vi "Unload Theme-Root Only.vi"(8 "Error In":errorcluster, 11 "Appearance Actor in":refnum<class "Appearance Actor.lvclass">) -> (0 "Error Out":errorcluster, 3 "Appearance Actor out":refnum<class "Appearance Actor.lvclass">)   [LabVIEW 2021, in "Appearance Actor.lvlib" / "Appearance Actor.lvclass"]
uses:
  Appearance Actor.lvclass
  C:/Program Files (x86)/National Instruments/LabVIEW 2021/vi.lib/ActorFramework/Actor/Actor.lvclass
  <vilib>/ActorFramework/Message Enqueuer/Message Enqueuer.lvclass
  <vilib>/ActorFramework/Actor/Actor.lvclass/Actor.ctl
  Appearance Actor.lvclass/Appearance Actor.ctl
  <vilib>/Utility/config.llb/Config Data RefNum.ctl
  <vilib>/ActorFramework/Actor/Actor.lvclass
  <vilib>/Utility/config.llb/NI_LVConfig.lvlib
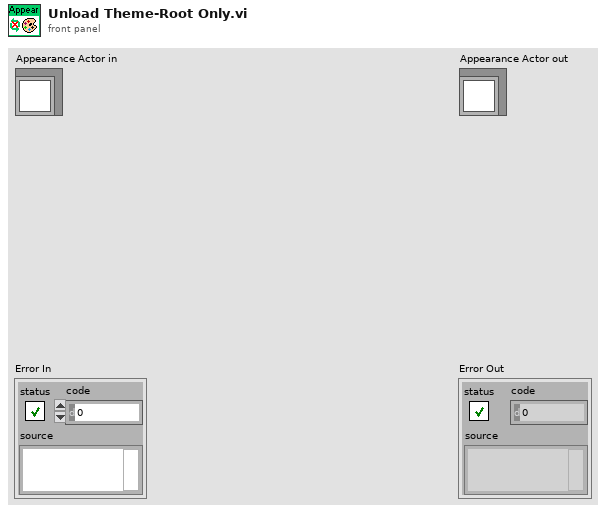
[diagram p1: front panel]
types:
  T1 = typedef "NI_LVConfig.lvlib/Config Data RefNum.ctl" = refnum<k1>
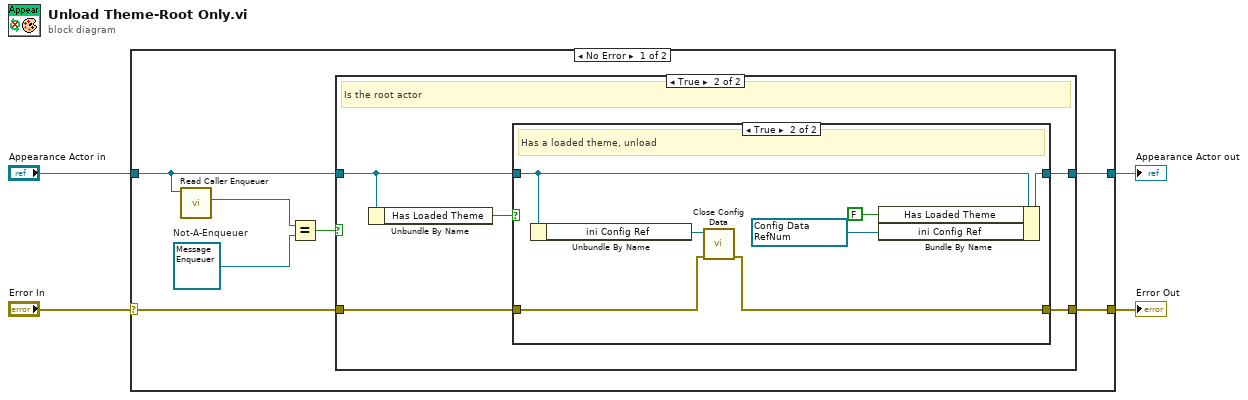
[diagram p0: block diagram]
diagram:
  n1 = case shown="No Error" "Error In" {
    selector: "Error In" -> [w6 w29]
    tunnel: [w5 w29] -> w3
    tunnel: [w7 w28] -> w1
    tunnel: "Appearance Actor in" -> [w8 w28]
    frame No Error {
      w10 = refnum<class "Message Enqueuer.lvclass"> refnum  # Not-A-Enqueuer
      n2 = call <vilib>:"Read Caller Enqueuer.vi"("Actor"=w8) -> ("Caller Enqueuer"=w11:refnum<class "Message Enqueuer.lvclass">)  [unwired: 10 in]
      n3 = Equal?(x=w11, y=w10) -> (x = y?=w9:bool)
      n4 = case shown="True" w9 {
        tunnel: w6 -> [w12 w17]
        tunnel: [w12 w16] -> w5
        tunnel: [w13 w18] -> w7
        tunnel: w8 -> [w13 w15]
        frame False {
          # "Is a nested actor"
        }
        frame True {
          # "Is the root actor"
          n5 = Unbundle By Name(w15) -> ("Has Loaded Theme"=w14:bool)
          n6 = case shown="True" w14 {
            tunnel: w15 -> [w20 w25]
            tunnel: [w20 w27] -> w18
            tunnel: w17 -> [w19 w23]
            tunnel: [w19 w22] -> w16
            frame False {
              # "No loaded theme"
            }
            frame True {
              w21 = T1 refnum items=["config data"] ("Theme Data.ini Config Ref")
              # "Has a loaded theme, unload"
              n7 = Unbundle By Name(w25) -> ("ini Config Ref"=w24:T1)
              n8 = call <vilib>:"Close Config Data.vi"("error in (no error)"=w23, "refnum"=w24) -> ("error out"=w22:errorcluster)  [unwired: 8 in, 1 out]
              n9 = Bundle By Name(cluster=w25, "Has Loaded Theme"=FALSE, "ini Config Ref"=w21) -> (w27:refnum<class "Appearance Actor.lvclass">)
            }
          }
        }
      }
    }
    frame Error {
    }
  }
  "Error Out" <- w3
  "Appearance Actor out" <- w1
